vi "IDN.vi"(8 "error in (no error)":errorcluster, 11 "refnum in":T1) -> (0 "error out":errorcluster, 2 "IDN out":string, 3 "refnum out":T1, 4 "question out":string="*IDN?")   [LabVIEW 2020, in "Korad KA3305P.lvlib"]
uses:
  Korad KA3305P.lvlib
  Reference.ctl
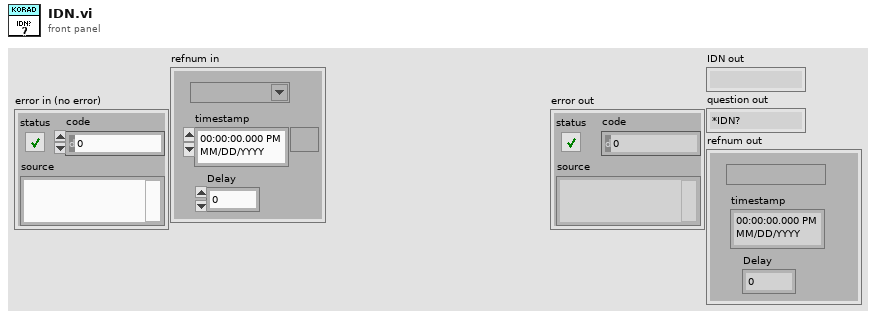
[diagram p1: front panel]
types:
  T1 = typedef "Korad KA3305P.lvlib/Reference.ctl" = cluster{"refnum":refnum<visa-resource-name>, "timestamp":timestamp, "Delay":dbl}
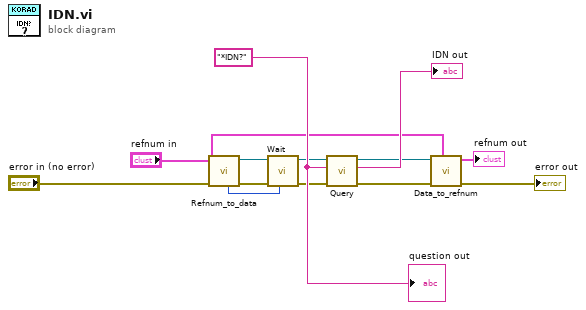
[diagram p0: block diagram]
diagram:
  w13 = "*IDN?" ("data in")
  n1 = call "Refnum_to_data.vi"("error in (no error)"="error in (no error)", "refnum in"="refnum in") -> ("error out"=w9:errorcluster, "DAQ refnum out"=w7:refnum<visa-resource-name>, "delay out"=w5:u32)  [unwired: 7 in]
  n2 = call "Wait.vi"("milliseconds to wait"=w5, "error in (no error)"=w9, "refnum in"=w7) -> ("error out"=w8:errorcluster, "refnum out"=w6:refnum<visa-resource-name>)  [unwired: 7 in]
  n3 = call "Query.vi"("error in (no error)"=w8, "data in"=w13, "refnum in"=w6) -> ("error out"=w11:errorcluster, "data out"=→"IDN out":string, "refnum out"=w3:refnum<visa-resource-name>)  [unwired: 6 in]
  n4 = call "Data_to_refnum.vi"("refnum in"="refnum in", "error in (no error)"=w11, "DAQ refnum in"=w3) -> ("error out"=→"error out":errorcluster, "refnum out"=→"refnum out":T1)  [unwired: 7 in]
  "question out" <- w13
